vi "Deembed S-parameters.vi"(7 "Deembedding Side":u16(ring) items=["Input", "Output"], 8 "error in (no error)":errorcluster, 10 "Deembedding S-par array in":cdb[][](array[numeric]), 11 "Original S-par array in":cdb[][](array[numeric])) -> (0 "error out":errorcluster, 3 "Deembedded S-par array out":cdb[][](array[numeric]))   [LabVIEW 2023, in "NI_HFNetworkAnalysis.lvlib"]
doc: "Deembedded two networks defined by their S-parameters.\n\nWhen the deembedding is performed at input side, transformation assumes that the even ports of deembedding network are connected to the odd ports of original network.\n\nWhen the deembedding is performed at output side, transformation assumes that the even ports of original network are connected to the odd ports of deembedding network.\n\nInput and output S-parameter array rows are defined as \n<b>(S11,S12,S13,S14,...,S21,S22,S23,S24,...,S31,S32,S33,S34,...,S41,S42,S43,S44,...)</b>\n\n<b>Known Limitations</b>\nTransformation supports only 2n-port networks."
uses:
  NI_HFNetworkAnalysis.lvlib
  <vilib>/Analysis/baseanly.llb/Complex A x B.vi
  <vilib>/Analysis/Matrix/Numeric/Conversions/Array To Matrix - CA2.vi
  <vilib>/Analysis/baseanly.llb/Complex Inverse Matrix.vi
  <vilib>/Analysis/Matrix/NI_Matrix.lvlib
  <vilib>/Analysis/NI_AALBase.lvlib
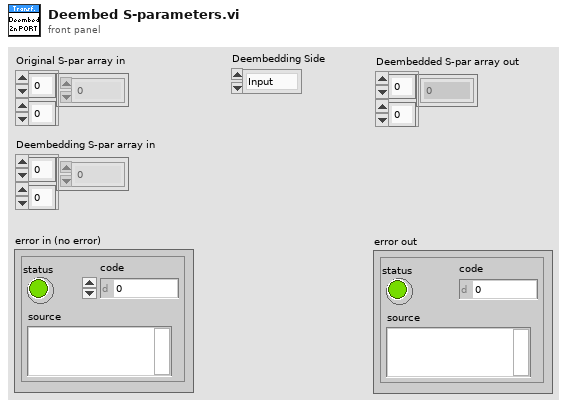
[diagram p1: front panel]
types:
  T1 = typedef "NI_Matrix.lvlib/ComplexMatrix.ctl" = cdb[][]
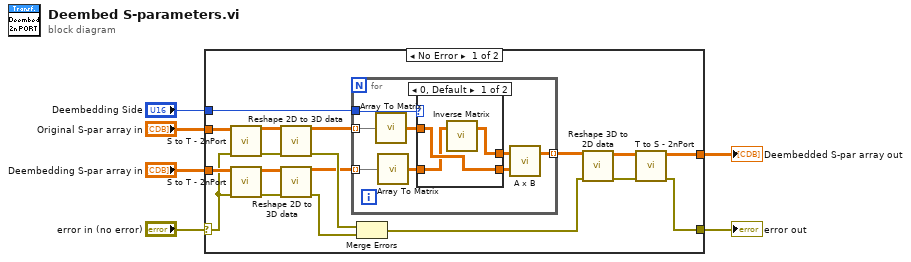
[diagram p0: block diagram]
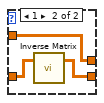
[diagram p2: hidden frame]
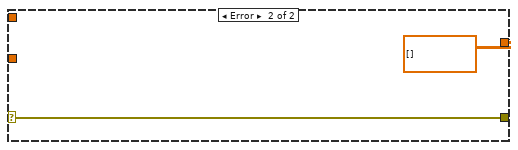
[diagram p3: hidden frame]
diagram:
  n1 = case shown="No Error" "error in (no error)" {
    selector: "error in (no error)" -> [w14 w40]
    tunnel: [w10 w40] -> w6
    tunnel: [w9 cdb[][] [] ("Parameters Out (2D)")] -> w5
    tunnel: "Deembedding S-par array in" -> [w24 _]
    tunnel: "Original S-par array in" -> [w23 _]
    tunnel: "Deembedding Side" -> [w7 _]
    frame No Error {
      n2 = call "S to T - 2nPort.vi"("error in (no error)"=w14, "S-par Array In"=w23) -> ("error out"=w20:errorcluster, "T-par Array Out"=w21:cdb[][])  [unwired: 8 in]
      n3 = call "S to T - 2nPort.vi"("error in (no error)"=w14, "S-par Array In"=w24) -> ("error out"=w19:errorcluster, "T-par Array Out"=w22:cdb[][])  [unwired: 8 in]
      n4 = call "Reshape 2D to 3D data.vi"("Parameters In (2D)"=w21, "Error In"=w20) -> ("Parameters Out (3D)"=w18:cdb[][][], "Error Out"=w12:errorcluster)  [unwired: 12 in]
      n5 = call "Reshape 2D to 3D data.vi"("Parameters In (2D)"=w22, "Error In"=w19) -> ("Parameters Out (3D)"=w8:cdb[][][], "Error Out"=w13:errorcluster)  [unwired: 12 in]
      n6 = for {
        tunnel: w18 -> [w32] mode=indexing
        tunnel: w8 -> [w31] mode=indexing
        tunnel: [w30] -> w17 mode=indexing
        tunnel: w7 -> [w29]
        n7 = call-poly <vilib>:"Array To Matrix.vi"("Complex 2D Array"=w32) -> ("Complex Matrix"=w26:T1)
        n8 = call-poly <vilib>:"Array To Matrix.vi"("Complex 2D Array"=w31) -> ("Complex Matrix"=w28:T1)
        n9 = case shown="0, Default" w29 {
          tunnel: w28 -> [w33 w38]
          tunnel: [w34 w37] -> w27
          tunnel: w26 -> [w34 w36]
          tunnel: [w35 w36] -> w25
          frame 0, Default {
            n10 = call-poly <vilib>:"Inverse Matrix.vi"("Input Matrix"=w33) -> ("Inverse Matrix"=w35:T1)  [unwired: 1 in, 1 out]
          }
          frame 1 {
            n11 = call-poly <vilib>:"Inverse Matrix.vi"("Input Matrix"=w38) -> ("Inverse Matrix"=w37:T1)  [unwired: 1 in, 1 out]
          }
        }
        n12 = call-poly <vilib>:"A x B.vi"("B"=w27, "A"=w25) -> ("A x B"=w30:T1)  [unwired: 1 out]
      }
      n13 = Merge Errors(w12, w13) -> (w11:errorcluster)
      n14 = call "Reshape 3D to 2D data.vi"("Parameters In (3D)"=w17, "Error In"=w11) -> ("Parameters Out (2D)"=w16:cdb[][], "Error Out"=w15:errorcluster)  [unwired: 12 in]
      n15 = call "T to S - 2nPort.vi"("error in (no error)"=w15, "T-par Array In"=w16) -> ("error out"=w10:errorcluster, "S-par Array Out"=w9:cdb[][])  [unwired: 8 in]
    }
    frame Error {
    }
  }
  "error out" <- w6
  "Deembedded S-par array out" <- w5
